vi "GUI_Mlink.vi"() -> ()   [LabVIEW 2020]
uses:
  Shared/GUI_Template/GUI_master/tcp_new_data_event.ctl
  Shared/GUI_Template/GUI_master/tcp new data cluster.ctl
panel:
  in  "Scale":T1(ring)
  in  "trigger::1":enum16{"Internal", "External"}(ring) caption="Trigger"
  in  "stop":bool
  in  "Select device":string(combo)="HPD_EnergyMeter"
  in  "data::1":dbl=25.5 caption="HPD Energy Meter (J)" min=0.0 max=300000000.0 format="%#_6p"
  out "GUIdevice 1":string="HPD_EnergyMeter"
  in  "Clear 2":bool
  out "Ch1":cluster{dbl[], dbl[]}(graph)
  out "Ch1 2":cluster{dbl[], dbl[]}(graph)
  out "tcp data event 2":T2
  out "validdata::1":enum16{"yes", "no"}(ring)
  in  "polarity::1":enum16{"Positive", "Negative"}(ring) caption="Trigger Signal Polarity"
  in  "autorange::1":enum16{"off", "on"}(ring) caption="AutoRange"
  in  "datastream::1":enum16{"off", "on"}(ring)
  in  "insert tag":bool=TRUE
  # "HPD Energy Meter"
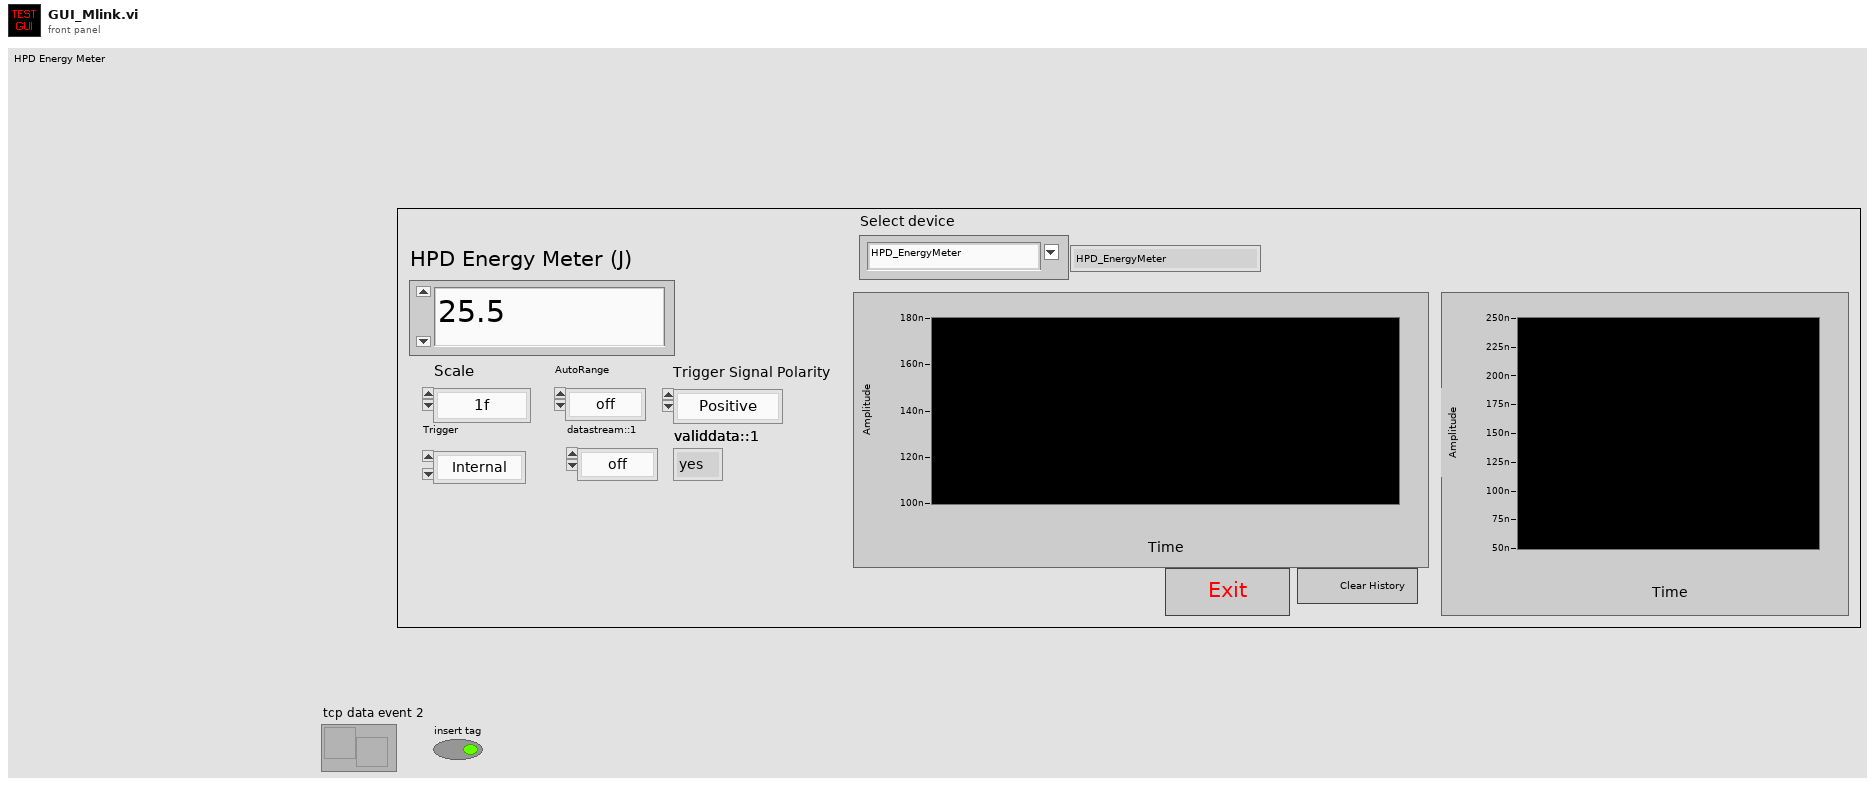
[diagram p1: front panel]
types:
  T1 = enum16{"1f", "3f", "10f", "30f", "100f", "300f", "1p", "3p", "10p", "30p", "100p", "300p", "1n", "3n", "10n", "30n", "100n", "300n", "1u", "3u", "10u", "30u", "100u", "300u", "1m", "3m", "10m", "30m", "100m", "300m", "1", "3", "10", "30", "100", "300", "1K", "3K", "10K", "30K", "100K", "300K", "1M", "3M", "10M", "30M", "100M", "300M"}
  T2 = typedef "tcp_new_data_event.ctl" = refnum<user-event>
  T3 = enum32{"invalid app kind", "Development System", "Run Time System", "Student Edition", "Embedded LabVIEW", "Evaluation", "Custom"}
  T4 = typedef "tcp new data cluster.ctl" = cluster{"EventEnum":enum16{"new data", "connection status update"}, "Device name":string}
  T5 = enum32{"Invalid", "Standard", "Closed", "Hidden", "Minimized", "Maximized"}
  T6 = cluster{"Core":cluster{"Current VI Reference":refnum<vi>, "Close Panel on Exit?":bool}, "Your Boolean data":bool, "Your string data":string, "SuperGUI":cluster{"STOP queue":refnum<queue>, "SuperGUI ref":refnum<vi>, "event reg":refnum<event-registration>}, "Timer":u32}
  T7 = cluster{"STOP queue":refnum<queue>, "SuperGUI ref":refnum<vi>, "event reg":refnum<event-registration>}
  T8 = cluster{"Current VI Reference":refnum<vi>, "Close Panel on Exit?":bool}
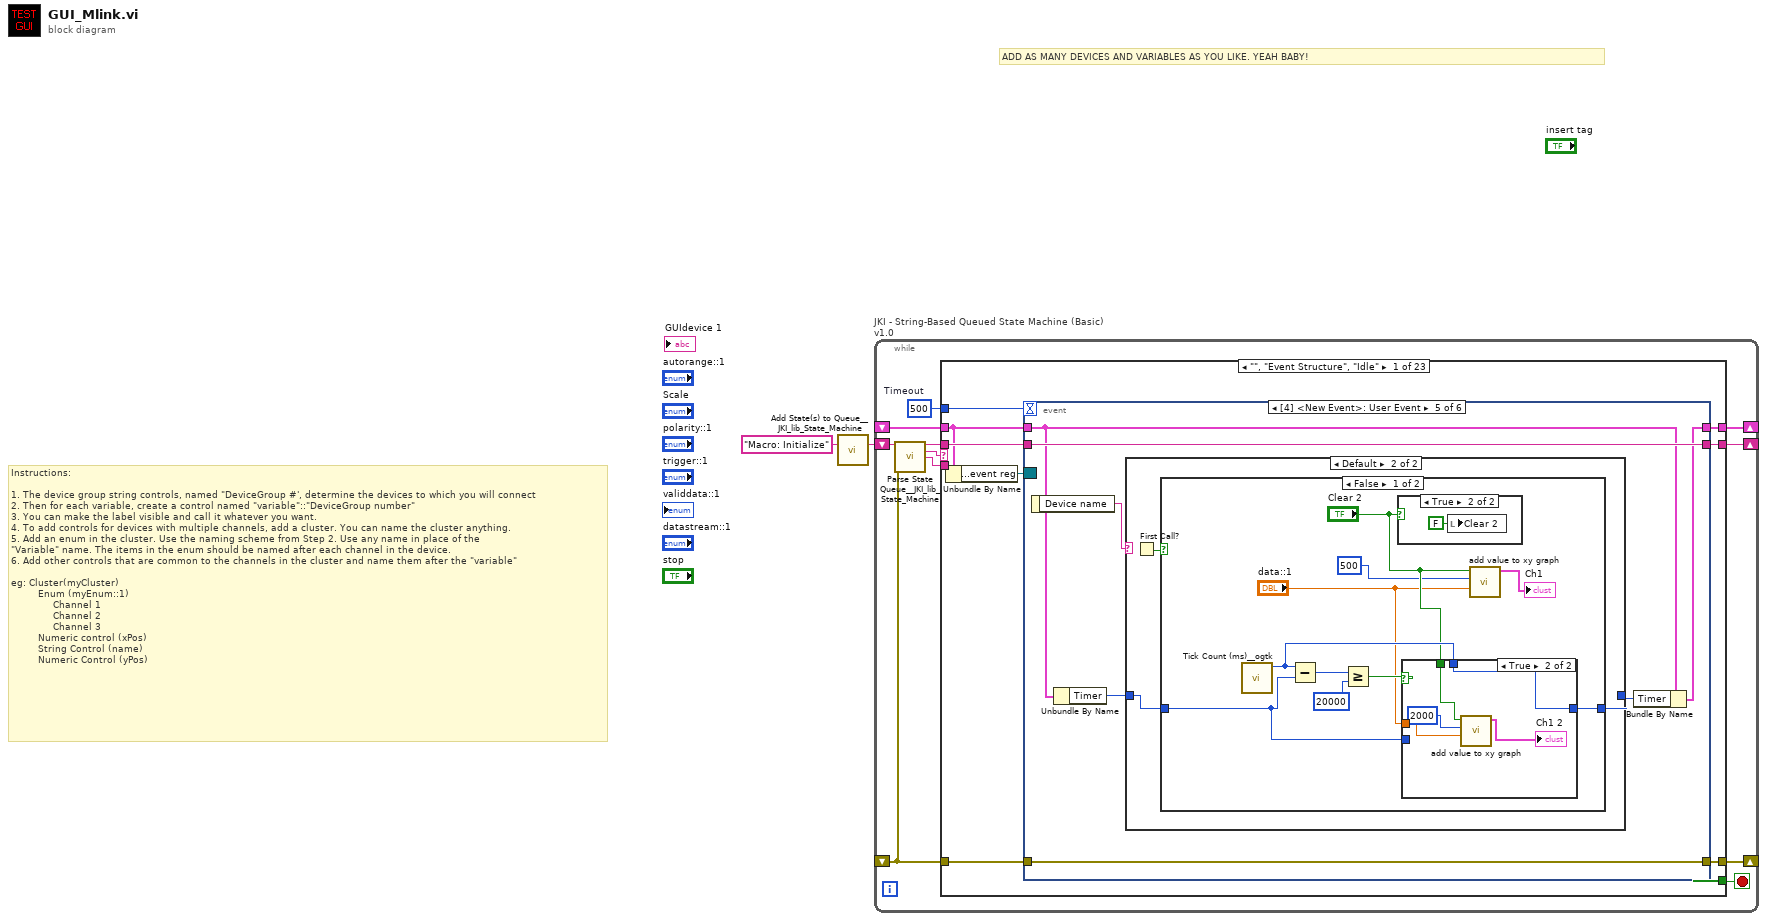
[diagram p0: block diagram]
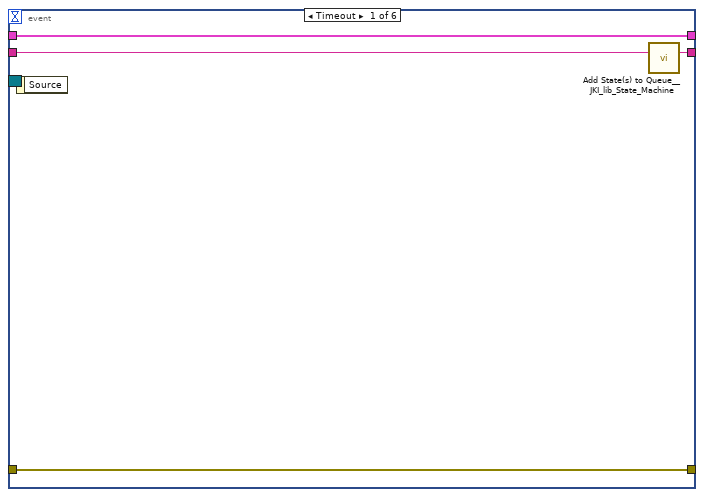
[diagram p2: hidden frame]
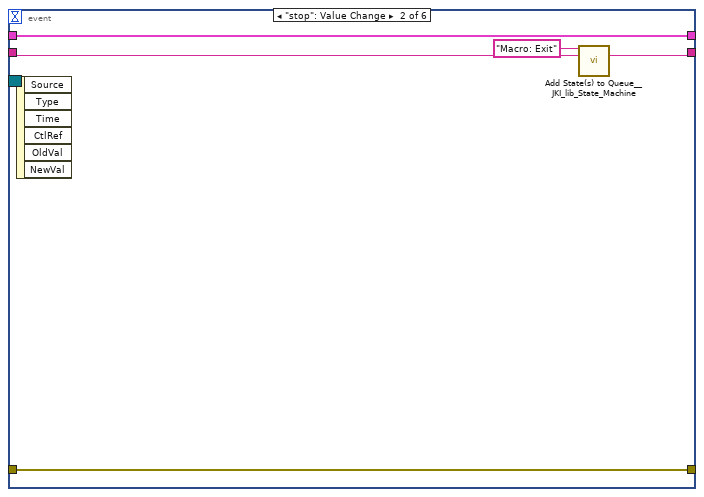
[diagram p3: hidden frame]
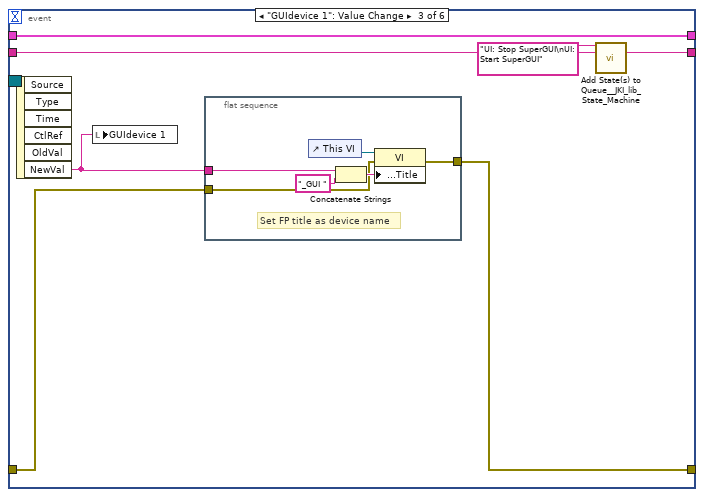
[diagram p4: hidden frame]
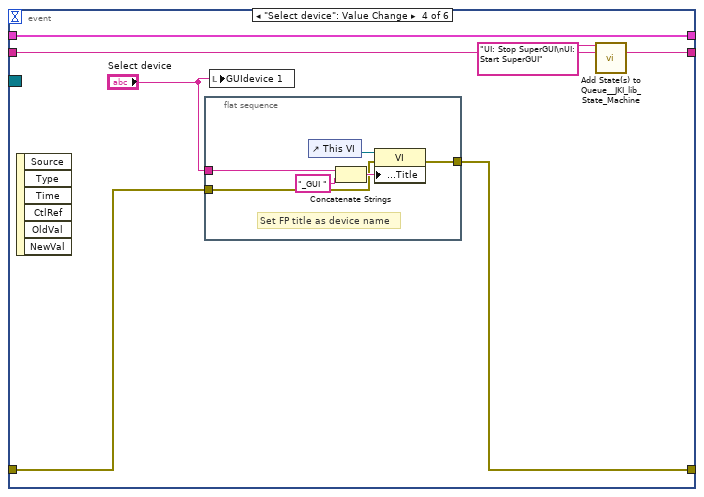
[diagram p5: hidden frame]
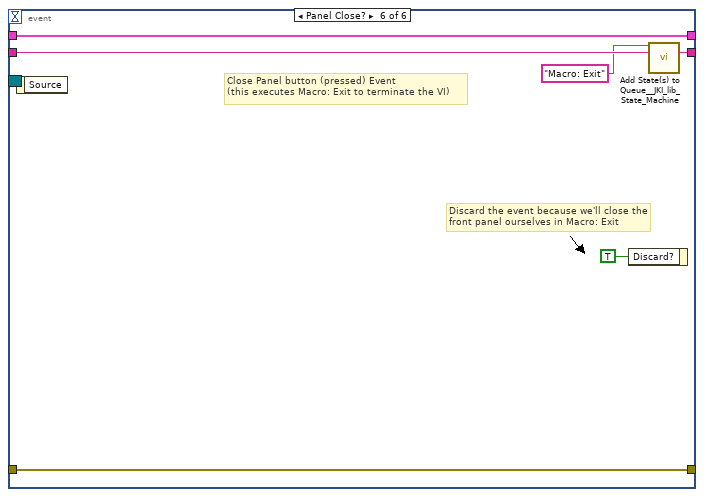
[diagram p10: hidden frame]
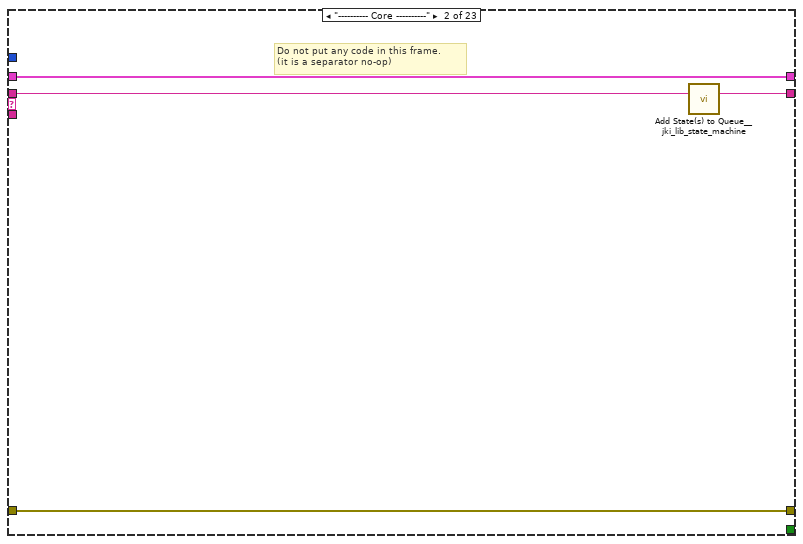
[diagram p11: hidden frame]
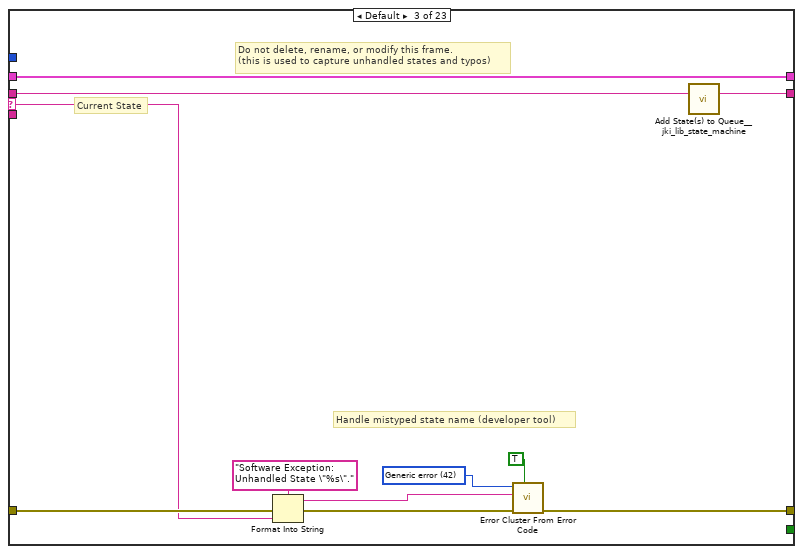
[diagram p12: hidden frame]
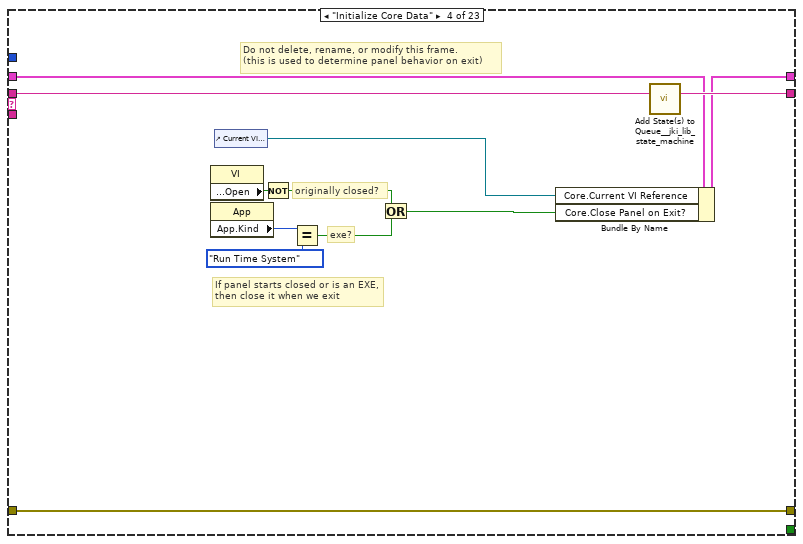
[diagram p13: hidden frame]
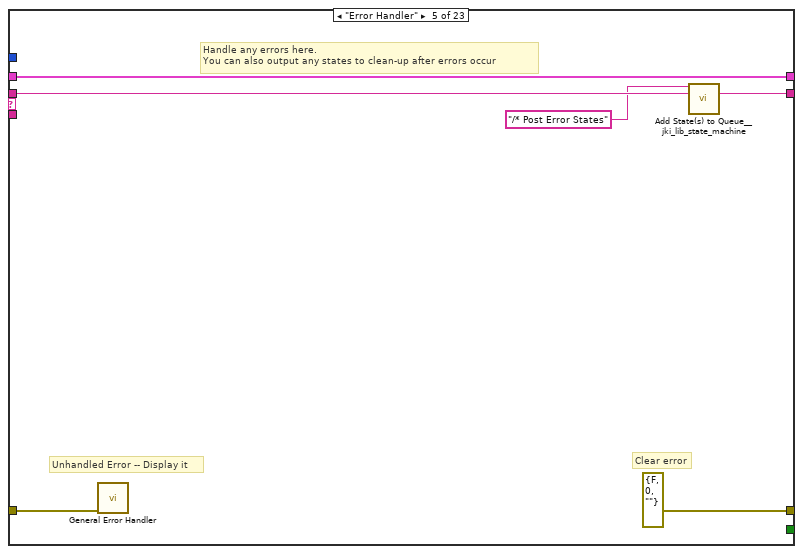
[diagram p14: hidden frame]
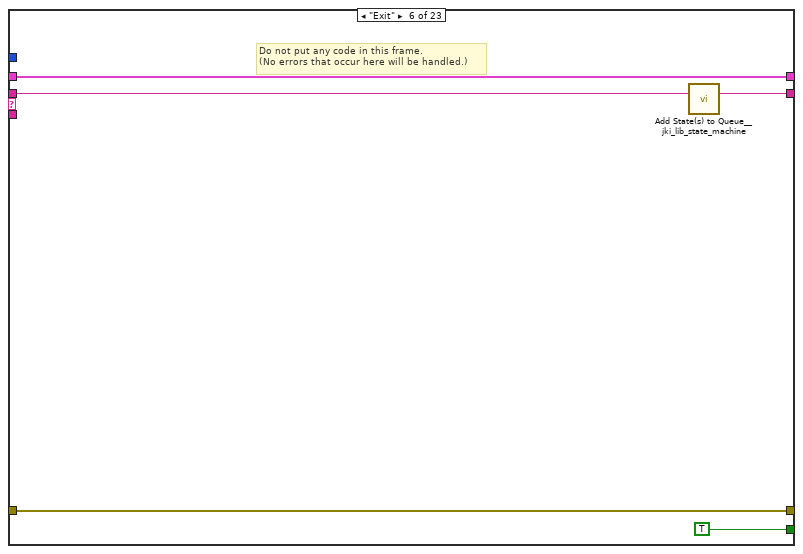
[diagram p15: hidden frame]
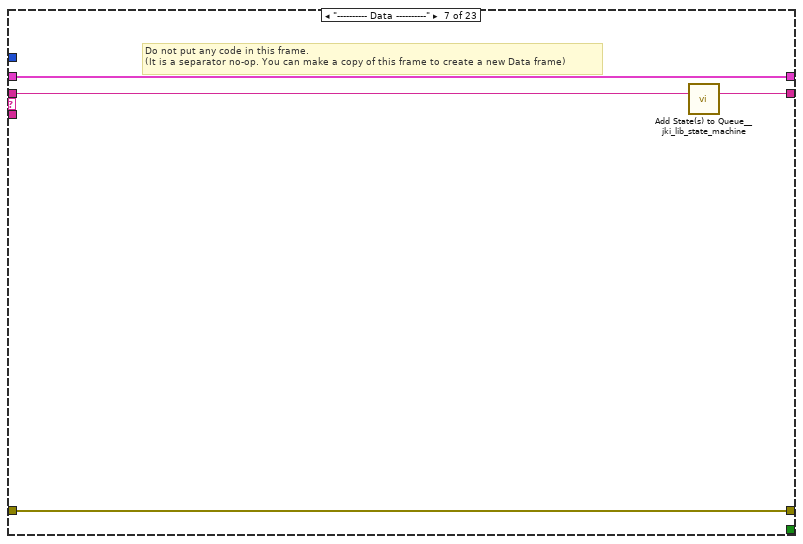
[diagram p16: hidden frame]
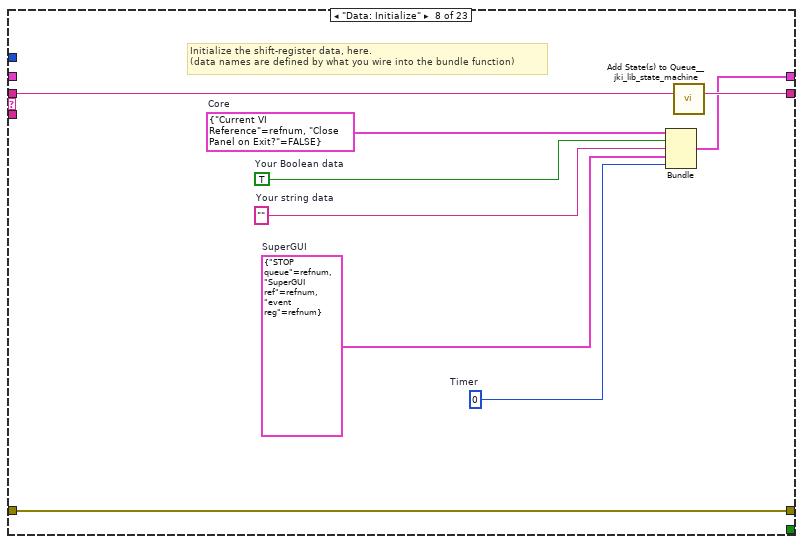
[diagram p17: hidden frame]
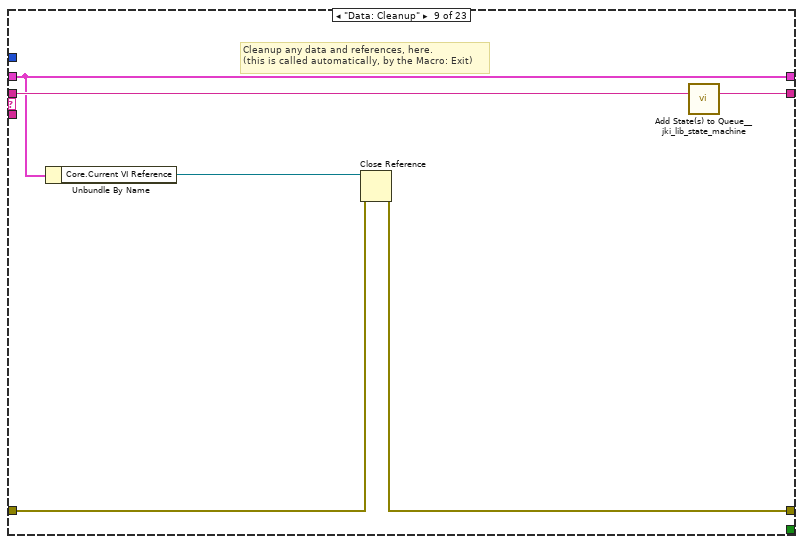
[diagram p18: hidden frame]
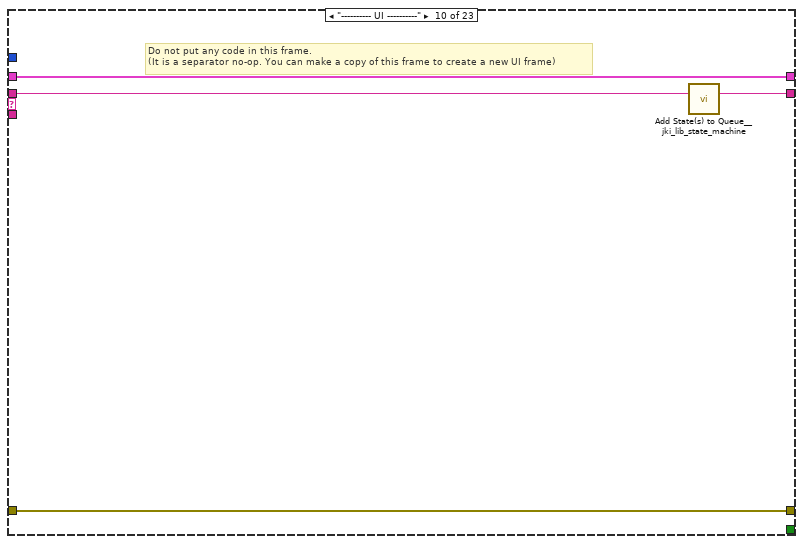
[diagram p19: hidden frame]
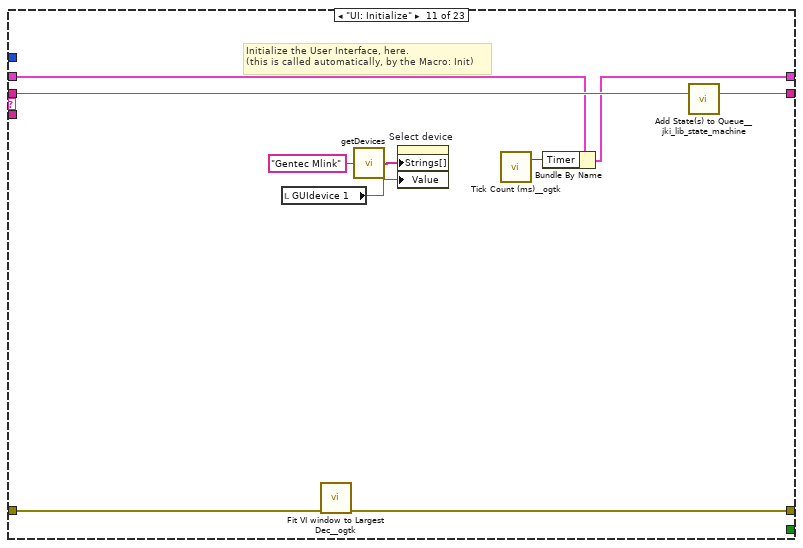
[diagram p20: hidden frame]
diagram:
  # "Instructions:\n\n1. The device group string controls, named \"DeviceGroup #', determine the devices to which you will connect\n2. Then for each variable, create a control named \"variable\"::\"DeviceGroup number\"\n3. You can make the label visible and call it whatever you want.\n4. To add controls for devices with multiple channels, add a cluster. You can name the cluster anything.\n5. Add an enum in the cluster. Use the naming scheme from Step 2. Use any name in place of the \n\"Variable\" name. The items in the enum should be named after each channel in the device. \n6. Add other controls that are common to the channels in the cluster and name them after the \"variable\"\n\neg: Cluster(myCluster)\n         Enum (myEnum::1)\n              Channel 1 \n              Channel 2\n              Channel 3\n         Numeric control (xPos)\n         String Control (name)\n         Numeric Control (yPos)"
  # "ADD AS MANY DEVICES AND VARIABLES AS YOU LIKE. YEAH BABY!"
  n1 = call <vilib>:"Add State(s) to Queue__JKI_lib_State_Machine.vi"("State(s) in (\"\")"="Macro: Initialize") -> ("States Out"=w2:string)  [unwired: 14 in]
  n2 = while "JKI - String-Based Queued State Machine (Basic) v1.0" {
    shift-right: [w6] -> _
    shift-left: _ -> [w5]
    shift-right: [w9] -> _
    shift-left: _ -> [w3]
    shift-right: [w8] -> _
    shift-left: w2 -> [w10]
    stop <- w7 stop-if-true
    w4 = 500  # Timeout
    n3 = call <vilib>:"Parse State Queue__JKI_lib_State_Machine.vi"("State Queue"=w10, "Error In (no error)"=w3) -> ("Remaining States"=w12:string, "Current State"=w13:string, "Arguments"=w11:string)  [unwired: 11 in]
    n4 = case shown="\"\", \"Event Structure\", \"Idle\"" w13 {
      selector: w13 -> [_ _ w96 _ _ _ _ _ _ _ _ _ _ _ _ _ _ _ _ _ _ _ _]
      tunnel: w12 -> [w21 w95 w100 w118 w124 w129 w133 w142 w148 w152 w162 w166 w172 w207 w215 w221 w232 w258 w263 w273 w277 w281 w285]
      tunnel: w11 -> [_ _ _ _ _ _ _ _ _ _ _ _ _ _ _ w216 w226 _ _ _ _ _ _]
      tunnel: w5 -> [w15 w92 w98 w109 w121 w127 w130 _ w143 w149 w155 w164 w170 w198 w210 w219 w228 w255 w260 w270 w274 w278 w282]
      tunnel: [w19 w93 w102 w115 errorcluster {"status"=FALSE, "code"=0, "source"=""} ("error out") w126 w131 w139 w144 w150 w159 w163 w167 w191 w208 w217 w229 w256 w261 w271 w275 w279 w283] -> w9
      tunnel: w3 -> [w18 w93 w101 w115 w120 w126 w131 w139 w145 w150 w160 w163 w168 w192 w209 w218 w230 w256 w261 w271 w275 w279 w283]
      tunnel: [w20 w94 w99 w117 w123 w128 w132 w141 w147 w151 w161 w165 w171 w206 w214 w220 w231 w257 w262 w272 w276 w280 w284] -> w8
      tunnel: [_ _ _ _ _ TRUE _ _ _ _ _ _ _ _ _ _ _ _ _ _ _ _ _] -> w7
      tunnel: [w17 w92 w98 w116 w121 w127 w130 w140 w143 w149 w154 w164 w170 w197 w210 w219 w228 w255 w260 w270 w274 w278 w282] -> w6
      tunnel: w4 -> [w16 _ _ _ _ _ _ _ _ _ _ _ _ _ _ _ _ _ _ _ _ _ _]
      frame "", "Event Structure", "Idle" {
        n5 = Unbundle By Name(w15) -> ("SuperGUI.event reg"=w14:refnum<event-registration>)
        n6 = event shown="[4] <New Event>: User Event" {
          selector: w14 -> [_ _ _ _ _ _]
          dyn-events: _ -> [_ _ _ _ _ _]
          timeout: w16 -> [_ _ _ _ _ _]
          tunnel: w21 -> [w25 w28 w34 w47 w63 w91]
          tunnel: [w24 w27 w33 w46 w63 w90] -> w20
          tunnel: w15 -> [w22 w30 w37 w50 w59 w88]
          tunnel: [w23 w29 w35 w48 w62 w89] -> w19
          tunnel: w18 -> [w23 w29 w36 w49 w62 w89]
          tunnel: [w22 w30 w37 w50 w58 w88] -> w17
          event Timeout {
            n7 = event-data() -> ()  [unwired: 1 in, 1 out]
            n8 = call <vilib>:"Add State(s) to Queue__JKI_lib_State_Machine.vi"("State(s) in (\"\")"=w25) -> ("States Out"=w24:string)  [unwired: 14 in]
          }
          event "stop": Value Change {
            n9 = event-data() -> ()  [unwired: 1 in, 6 out]
            n10 = call <vilib>:"Add State(s) to Queue__JKI_lib_State_Machine.vi"("State(s) in Front (\"\")"="Macro: Exit", "State(s) in (\"\")"=w28) -> ("States Out"=w27:string)  [unwired: 13 in]
          }
          event "GUIdevice 1": Value Change {
            n11 = event-data() -> ("NewVal"=w31:string)  [unwired: 1 in, 5 out]
            n12 = local write "GUIdevice 1"(w31) -> ()
            n13 = flat-sequence {
              tunnel: [w40] -> w35
              tunnel: w36 -> [w39]
              tunnel: w31 -> [w38]
              frame #0 {
                # "Set FP title as device name"
                n14 = control-ref of="This VI"() -> (w43:refnum<vi>)
                n15 = Concatenate Strings(w38, "_GUI ") -> (w42:string)
                n16 = property class="VI"(reference=w43, error in=w39, "Front Panel.Title"=w42) -> (error out=w40:errorcluster)  [unwired: 1 out]
              }
            }
            n17 = call <vilib>:"Add State(s) to Queue__JKI_lib_State_Machine.vi"("State(s) in Front (\"\")"="UI: Stop SuperGUI\nUI: Start SuperGUI", "State(s) in (\"\")"=w34) -> ("States Out"=w33:string)  [unwired: 13 in]
          }
          event "Select device": Value Change {
            n18 = event-data() -> ()  [unwired: 1 in, 6 out]
            n19 = flat-sequence {
              tunnel: [w53] -> w48
              tunnel: w49 -> [w52]
              tunnel: "Select device" -> [w51]
              frame #0 {
                # "Set FP title as device name"
                n20 = control-ref of="This VI"() -> (w56:refnum<vi>)
                n21 = Concatenate Strings(w51, "_GUI ") -> (w55:string)
                n22 = property class="VI"(reference=w56, error in=w52, "Front Panel.Title"=w55) -> (error out=w53:errorcluster)  [unwired: 1 out]
              }
            }
            n23 = local write "GUIdevice 1"("Select device") -> ()
            n24 = call <vilib>:"Add State(s) to Queue__JKI_lib_State_Machine.vi"("State(s) in Front (\"\")"="UI: Stop SuperGUI\nUI: Start SuperGUI", "State(s) in (\"\")"=w47) -> ("States Out"=w46:string)  [unwired: 13 in]
          }
          event User Event {
            n25 = event-data() -> ("Device name"=w60:string)  [unwired: 1 in]
            n26 = Unbundle By Name(w59) -> ("Timer"=w61:u32)
            n27 = case shown="Default" w60 {
              tunnel: w61 -> [w64 w65]
              tunnel: [w64 w66] -> w57
              frame "" {
              }
              frame Default {
                n28 = First Call?() -> (First Call?: T/F=w67:bool)
                n29 = case shown="False" w67 {
                  tunnel: w65 -> [w72 w85]
                  tunnel: [w74 w85] -> w66
                  frame False {
                    n30 = call <userlib>:"Tick Count (ms)__ogtk.vi"() -> ("millisecond timer value"=w73:u32)  [unwired: 10 in, 1 out]
                    n31 = Subtract(x=w73, y=w72) -> (x-y=w76:u32)
                    n32 = Greater Or Equal?(x=w76, y=u32 20000 ("min time between updates")) -> (x >= y?=w75:bool)
                    n33 = case shown="True" "Clear 2" {
                      frame False {
                      }
                      frame True {
                        n34 = local write "Clear 2"(FALSE ("Clear")) -> ()
                      }
                    }
                    n35 = case shown="True" w75 {
                      tunnel: "data::1" -> [_ w81]
                      tunnel: [w78 w83] -> w74
                      tunnel: w73 -> [_ w83]
                      tunnel: w72 -> [w78 _]
                      tunnel: "Clear 2" -> [_ w79]
                      frame False {
                      }
                      frame True {
                        n36 = call "add value to xy graph.vi"("new value"=w81, "max points"=2000, "Wire in Stop To Clear Graph on Each Run"=w79) -> ("XY Graph"=→"Ch1 2":cluster{dbl[], dbl[]})  [unwired: 8 in]
                      }
                    }
                    n37 = call "add value to xy graph.vi"("new value"="data::1", "max points"=500, "Wire in Stop To Clear Graph on Each Run"="Clear 2") -> ("XY Graph"=→"Ch1":cluster{dbl[], dbl[]})  [unwired: 8 in]
                  }
                  frame True {
                  }
                }
              }
            }
            n38 = Bundle By Name(cluster=w59, "Timer"=w57) -> (w58:T6)
          }
          event Panel Close? {
            # "Discard the event because we'll close the front panel ourselves in Macro: Exit"
            # "Close Panel button (pressed) Event\n(this executes Macro: Exit to terminate the VI)"
            n39 = event-data() -> ()  [unwired: 1 in, 1 out]
            n40 = event-data("Discard?"=TRUE) -> ()  [unwired: 1 in, 1 out]
            n41 = call <vilib>:"Add State(s) to Queue__JKI_lib_State_Machine.vi"("State(s) in Front (\"\")"="Macro: Exit", "State(s) in (\"\")"=w91) -> ("States Out"=w90:string)  [unwired: 13 in]
          }
        }
      }
      frame "---------- Core ----------" {
        # "Do not put any code in this frame.\n(it is a separator no-op)"
        n42 = call <vilib>:"Add State(s) to Queue__jki_lib_state_machine.vi"("State(s) in (\"\")"=w95) -> ("States Out"=w94:string)  [unwired: 14 in]
      }
      frame Default {
        w105 = 42 items=["No error", "Argument error", "Memory is full", "Out of zone", "End of file", "File already open", "Generic file I/O error", "File not found", "File permission error", "Disk is full", "Duplicate path", "Too many files open", "System feature not enabled", "Resource file not found", "Cannot add resource", "Resource not found", "Image not found", "Image memory error", "Pen does not exist", "Config type invalid", "Config token not found", "Config parse error", "Config memory error", "Bad external code format", "Bad external code offset", "External code not present", "Null window", "Destroy window error", "Null menu", "Print aborted", "Bad print record", "Print driver error", "Windows error during printing", "Memory error during printing", "Print dialog error", "Generic print error", "Invalid device refnum", "Device not found", "Device parameter error", "Device unit error", "Cannot open device", "Device call aborted", "Generic error", "Cancelled by user", "Object ID too low", "Object ID too high", "Object not in heap", "Unknown heap", "Unknown object (invalid DefProc)", "Unknown object (DefProc not in table)", "Message out of range", "Invalid (null) method", "Unknown message", "Manager call not supported", "Bad address", "Network operation in progress", "Network operation timed out", "Connection is busy", "Network attribute not supported", "Network error", "Address in use", "System out of memory", "Connection aborted", "Connection refused", "Not connected", "Already connected", "Connection closed", "Initialization error (interapplication manager)", "Bad occurrence", "Wait on unbound occurrence handler", "Occurrence queue overflow", "Datalog type conflict", "Unused", "Unrecognized type (interapplication manager)", "Memory corrupt", "Failed to make temporary DLL", "Old CIN version", "Drag socket not found", "Failed to load drop-object", "Failed to register OLE object", "Failed to release OLE object", "Format specifier type mismatch", "Unknown format specifier", "Too few format specifiers", "Too many format specifiers", "Scan failed", "Newer CIN version", "Error converting to variant", "Runtime menu error", "Password tampered", "Variant attribute not found", "Incompatible variant data type", "Event data is not available", "Event Store is not present", "Occurrence is not found", "Event Queue is not created", "Event info is not available", "Refnum passed is NULL", "Error retrieving Class GUID", "Error retrieving CoClass GUID", "Error retrieving TypeLib GUID.", "Bad built application magic bytes.", "Specific driver is different from the specific driver associated with the Logical Name.", "There is no session opened to the class driver.", "Max Error", "MAX - Error with config objects", "MAX - Error loading configuration", "MAX - Group not supported"]
        # "Current State"
        # "Do not delete, rename, or modify this frame.\n(this is used to capture unhandled states and typos)"
        # "Handle mistyped state name (developer tool)"
        n43 = Format Into String(format string="Software Exception: Unhandled State \"%s\"." ("message"), error in=w101, w96) -> (resulting string=w104:string, error out=w103:errorcluster)  [unwired: 1 in]
        n44 = call <vilib>:"Error Cluster From Error Code.vi"("show call chain? (False)"=TRUE, "error in (no error)"=w103, "error message (\"\")"=w104, "error code (0)"=w105) -> ("error out"=w102:errorcluster)  [unwired: 5 in]
        n45 = call <vilib>:"Add State(s) to Queue__jki_lib_state_machine.vi"("State(s) in (\"\")"=w100) -> ("States Out"=w99:string)  [unwired: 14 in]
      }
      frame "Initialize Core Data" {
        # "Do not delete, rename, or modify this frame.\n(this is used to determine panel behavior on exit)"
        # "originally closed?"
        # "exe?"
        # "If panel starts closed or is an EXE, then close it when we exit"
        n46 = property class="VI"() -> ("Front Panel.Open"=w114:bool)  [unwired: 2 in, 2 out]
        n47 = property class="App"() -> ("App.Kind"=w113:T3)  [unwired: 2 in, 2 out]
        n48 = control-ref of="Current VI Reference"() -> (w107:refnum<vi>)
        n49 = Not(x=w114) -> (.not. x?=w111:bool)
        n50 = Equal?(x=w113, y=T3."Run Time System" ("Application:Kind")) -> (x = y?=w110:bool)
        n51 = Or(x=w111, y=w110) -> (x .or. y?=w108:bool)
        n52 = Bundle By Name(cluster=w109, "Core.Current VI Reference"=w107, "Core.Close Panel on Exit?"=w108) -> (w116:T6)
        n53 = call <vilib>:"Add State(s) to Queue__jki_lib_state_machine.vi"("State(s) in (\"\")"=w118) -> ("States Out"=w117:string)  [unwired: 14 in]
      }
      frame "Error Handler" {
        # "Unhandled Error -- Display it"
        # "Handle any errors here.\nYou can also output any states to clean-up after errors occur"
        # "Clear error"
        n54 = call <vilib>:"General Error Handler.vi"("error in (no error)"=w120) -> ()  [unwired: 10 in, 5 out]
        n55 = call <vilib>:"Add State(s) to Queue__jki_lib_state_machine.vi"("State(s) in Front (\"\")"="/* Post Error States", "State(s) in (\"\")"=w124) -> ("States Out"=w123:string)  [unwired: 13 in]
      }
      frame "Exit" {
        # "Do not put any code in this frame.\n(No errors that occur here will be handled.)"
        n56 = call <vilib>:"Add State(s) to Queue__jki_lib_state_machine.vi"("State(s) in (\"\")"=w129) -> ("States Out"=w128:string)  [unwired: 14 in]
      }
      frame "---------- Data ----------" {
        # "Do not put any code in this frame.\n(It is a separator no-op. You can make a copy of this frame to create a new Data frame)"
        n57 = call <vilib>:"Add State(s) to Queue__jki_lib_state_machine.vi"("State(s) in (\"\")"=w133) -> ("States Out"=w132:string)  [unwired: 14 in]
      }
      frame "Data: Initialize" {
        w134 = u32 0  # Timer
        w135 = T7 {"STOP queue"=refnum, "SuperGUI ref"=refnum, "event reg"=refnum}  # SuperGUI
        w136 = T8 {"Current VI Reference"=refnum, "Close Panel on Exit?"=FALSE}  # Core
        w138 = TRUE  # Your Boolean data
        w137 = ""  # Your string data
        # "Initialize the shift-register data, here.\n(data names are defined by what you wire into the bundle function)"
        n58 = Bundle("Core"=w136, "Your Boolean data"=w138, "Your string data"=w137, "SuperGUI"=w135, "Timer"=w134) -> (w140:T6)  [unwired: 1 in]
        n59 = call <vilib>:"Add State(s) to Queue__jki_lib_state_machine.vi"("State(s) in (\"\")"=w142) -> ("States Out"=w141:string)  [unwired: 14 in]
      }
      frame "Data: Cleanup" {
        # "Cleanup any data and references, here.\n(this is called automatically, by the Macro: Exit)"
        n60 = Unbundle By Name(w143) -> ("Core.Current VI Reference"=w146:refnum<vi>)
        n61 = Close Reference(reference=w146, error in (no error)=w145) -> (error out=w144:errorcluster)
        n62 = call <vilib>:"Add State(s) to Queue__jki_lib_state_machine.vi"("State(s) in (\"\")"=w148) -> ("States Out"=w147:string)  [unwired: 14 in]
      }
      frame "---------- UI ----------" {
        # "Do not put any code in this frame.\n(It is a separator no-op. You can make a copy of this frame to create a new UI frame)"
        n63 = call <vilib>:"Add State(s) to Queue__jki_lib_state_machine.vi"("State(s) in (\"\")"=w152) -> ("States Out"=w151:string)  [unwired: 14 in]
      }
      frame "UI: Initialize" {
        # "Initialize the User Interface, here.\n(this is called automatically, by the Macro: Init)"
        n64 = local read "GUIdevice 1"() -> (w156:string)
        n65 = call <userlib>:"Fit VI window to Largest Dec__ogtk.vi"("error in (no error)"=w160) -> ("error out"=w159:errorcluster)  [unwired: 5 in, 1 out]
        n66 = call "getDevices.vi"("Device Class"="Gentec Mlink") -> ("All Devices"=w158:string[])
        n67 = property on="Select device" class="CmbBox"("Strings[]"=w158, "Value"=w156) -> ()  [unwired: 2 in, 2 out]
        n68 = call <userlib>:"Tick Count (ms)__ogtk.vi"() -> ("millisecond timer value"=w153:u32)  [unwired: 10 in, 1 out]
        n69 = Bundle By Name(cluster=w155, "Timer"=w153) -> (w154:T6)
        n70 = call <vilib>:"Add State(s) to Queue__jki_lib_state_machine.vi"("State(s) in (\"\")"=w162) -> ("States Out"=w161:string)  [unwired: 14 in]
      }
      frame "UI: Update Device List" {
        n71 = call <vilib>:"Add State(s) to Queue__jki_lib_state_machine.vi"("State(s) in (\"\")"=w166) -> ("States Out"=w165:string)  [unwired: 14 in]
      }
      frame "UI: Get Device Name" {
        n72 = First Call?() -> (First Call?: T/F=w169:bool)
        n73 = case shown="True" w169 {
          tunnel: w168 -> [w173 w175]
          tunnel: [w173 w174] -> w167
          frame False {
          }
          frame True {
            n74 = disable-structure "Get Device name from control for vi mode\nand command line arg for exe" shown="RUN_TIME_ENGINE==True" {
              disable-tunnel: w175 -> [_ w177]
              disable-tunnel: [_ w176] -> w174
              frame condition #0 (active) {
              }
              frame condition #1 {
                n75 = control-ref of="This Application"() -> (w185:refnum<vi>)
                n76 = property class="App"(reference=w185) -> ("App.Args"=w184:string[])  [unwired: 1 in, 2 out]
                n77 = Index Array(array=w184, index #1=1 ("index")) -> (element #1=w178:string)  [unwired: 2 in, 2 out]
                n78 = Empty String/Path?(string/path=w178) -> (empty?=w182:bool)
                n79 = control-ref of="This VI"() -> (w181:refnum<vi>)
                n80 = case shown="False" w182 {
                  tunnel: w178 -> [w186 _]
                  frame False {
                    n81 = local write "GUIdevice 1"(w186) -> ()
                  }
                  frame True {
                  }
                }
                n82 = Concatenate Strings(w178, "_GUI ") -> (w180:string)
                n83 = property class="VI"(reference=w181, error in=w177, "Front Panel.Title"=w180) -> (error out=w176:errorcluster)  [unwired: 1 out]
              }
            }
          }
        }
        n84 = call <vilib>:"Add State(s) to Queue__jki_lib_state_machine.vi"("State(s) in (\"\")"=w172) -> ("States Out"=w171:string)  [unwired: 14 in]
      }
      frame "UI: Start SuperGUI" {
        # "create stop queue for supergui and its clones"
        # "x100 abort will be dependent on caller VI\nx80 abort will be independent of caller vi, this will abort vi when labview is closed."
        # "Start SuperGUI asynchronous way"
        n85 = vi-ref "GUI_Master_subvi_reentrant_queues.vi"() -> (w190:refnum<vi>)
        n86 = property class="VI"(reference=w190) -> ("Path"=w189:path)  [unwired: 1 in, 2 out]
        n87 = Create User Event(user event datatype=T4 {"EventEnum"=enum."new data", "Device name"="Device name"} ("New Event"), error in=w192) -> (user event=w193:refnum<user-event>, error out=w199:errorcluster)
        "tcp data event 2" <- w193
        n88 = control-ref of="This Application"() -> (w196:refnum<vi>)
        n89 = control-ref of="This VI"() -> (w195:refnum<vi>)
        n90 = Open VI Reference(type specifier VI Refnum (for type only)=refnum<vi> refnum, vi path=w189, options=256) -> (vi reference=w205:refnum<vi>, error out=w204:errorcluster)  [unwired: 3 in]
        n91 = register-events(w193) -> (reference out=w187:refnum<event-registration>)  [unwired: 2 in, 1 out]
        n92 = call "supergui create stop queue.vi"() -> ("STOP Queue out"=w201:refnum<queue>)  [unwired: 11 in]
        n93 = Current VI's Menubar() -> (w194:refnum<k9>)
        n94 = call-by-ref "Start Asynchronous Call"(reference=w205, error in=w204, "STOP Queue in"=w201, "This Application"=w196, 8:"error in (no error)"=w199, "tcp data event"=w193, "Caller menu reference"=w194, "Caller VI ref"=w195) -> (reference out=w188:refnum<vi>, error out=w191:errorcluster)  [unwired: 5 in, 1 out]
        n95 = Bundle By Name(cluster=w198, "SuperGUI.event reg"=w187, "SuperGUI.SuperGUI ref"=w188, "SuperGUI.STOP queue"=w201) -> (w197:T6)
        n96 = call <vilib>:"Add State(s) to Queue__jki_lib_state_machine.vi"("State(s) in (\"\")"=w207) -> ("States Out"=w206:string)  [unwired: 14 in]
      }
      frame "UI: Stop SuperGUI" {
        # "Stop Supergui Clone and wait until it exit properly"
        n97 = Unbundle By Name(w210) -> ("SuperGUI.SuperGUI ref"=w212:refnum<vi>, "SuperGUI.STOP queue"=w211:refnum<queue>)
        n98 = Release Queue(queue=w211, error in (no error)=w209) -> (error out=w213:errorcluster)  [unwired: 1 in, 2 out]
        n99 = call-by-ref "Wait On Asynchronous Call"(reference=w212, error in=w213) -> ("error out"=w208:errorcluster)  [unwired: 11 in, 2 out]
        n100 = call <vilib>:"Add State(s) to Queue__jki_lib_state_machine.vi"("State(s) in (\"\")"=w215) -> ("States Out"=w214:string)  [unwired: 14 in]
      }
      frame "UI: Cursor Set" {
        # "Argument"
        # "Set and Unset Cursor Busy.\n(Usage: \"UI: Cursor Set >> Busy|Idle\")"
        n101 = case shown="\"Idle\", Default" w216 {
          tunnel: w218 -> [w223 w225]
          tunnel: [w222 w224] -> w217
          frame "Idle", Default {
            n102 = call <vilib>:"Unset Busy.vi"("error in (no error)"=w223) -> ("error out"=w222:errorcluster)  [unwired: 10 in]
          }
          frame "Busy" {
            n103 = call <vilib>:"Set Busy.vi"("error in (no error)"=w225) -> ("error out"=w224:errorcluster)  [unwired: 9 in, 1 out]
          }
        }
        n104 = call <vilib>:"Add State(s) to Queue__jki_lib_state_machine.vi"("State(s) in (\"\")"=w221) -> ("States Out"=w220:string)  [unwired: 14 in]
      }
      frame "UI: Front Panel State" {
        # "Argument"
        # "Set Front Panel Open or Closed\n(Usage: \"UI: Front Panel State >> Open|Close\")"
        n105 = Unbundle By Name(w228) -> ("Core.Current VI Reference"=w227:refnum<vi>)
        n106 = case shown="\"Open\", Default" w226 {
          tunnel: w230 -> [w236 w249]
          tunnel: [w238 w250] -> w229
          tunnel: w227 -> [w237 w247]
          frame "Open", Default {
            n107 = property class="VI"(reference=w237, error in=w236) -> (reference out=w234:refnum<vi>, error out=w235:errorcluster, "Front Panel.Open"=w233:bool)
            n108 = case shown="False" w233 {
              tunnel: [w241 w244] -> w238
              tunnel: w235 -> [w240 w244]
              tunnel: w234 -> [w239 _]
              frame False {
                n109 = invoke class="VI" method="FP.Open"(reference=w239, error in=w240, "Activate"=TRUE, "State"=T5."Standard") -> (error out=w241:errorcluster)  [unwired: 1 in, 4 out]
              }
              frame True {
              }
            }
          }
          frame "Close" {
            n110 = property class="VI"(reference=w247, error in=w249) -> (reference out=w246:refnum<vi>, error out=w248:errorcluster, "Front Panel.Open"=w245:bool)
            n111 = case shown="True" w245 {
              tunnel: [w251 w254] -> w250
              tunnel: w248 -> [w251 w253]
              tunnel: w246 -> [_ w252]
              frame False {
              }
              frame True {
                n112 = invoke class="VI" method="FP.Close"(reference=w252, error in=w253) -> (error out=w254:errorcluster)  [unwired: 1 in, 2 out]
              }
            }
          }
        }
        n113 = call <vilib>:"Add State(s) to Queue__jki_lib_state_machine.vi"("State(s) in (\"\")"=w232) -> ("States Out"=w231:string)  [unwired: 14 in]
      }
      frame "---------- Macro ----------" {
        # "Do not put any code in this frame.\n(It is a separator no-op. You can make a copy of this frame to create a new Macro frame)"
        n114 = call <vilib>:"Add State(s) to Queue__jki_lib_state_machine.vi"("State(s) in (\"\")"=w258) -> ("States Out"=w257:string)  [unwired: 14 in]
      }
      frame "Macro: Initialize" {
        # "Initialization Macro\n(This is called once, when the VI starts)"
        n115 = call <vilib>:"Add State(s) to Queue__jki_lib_state_machine.vi"("State(s) in Front (\"\")"="Data: Initialize\nInitialize Core Data\nUI: Initialize\nUI: Update Device List\nUI: Get Device Name\nUI: Start SuperGUI\nUI: Front Panel State >> Open", "State(s) in (\"\")"=w263) -> ("States Out"=w262:string)  [unwired: 13 in]
      }
      frame "Macro: Exit" {
        # "Exit Macro\n(This is called once, when the VI exits)"
        n116 = Unbundle By Name(w270) -> ("Core.Close Panel on Exit?"=w269:bool)
        n117 = Select(t="UI: Front Panel State >> Close", s=w269, f="") -> (s? t:f=w266:string)
        n118 = call <vilib>:"Add State(s) to Queue__jki_lib_state_machine.vi"("State(s) in (\"\")"=w266, "State(s) at Back (\"\")"="Data: Cleanup\nExit") -> ("States Out"=w264:string)  [unwired: 13 in]
        n119 = call <vilib>:"Add State(s) to Queue__jki_lib_state_machine.vi"("State(s) in Front (\"\")"=w264, "State(s) in (\"\")"=w273) -> ("States Out"=w272:string)  [unwired: 13 in]
      }
      frame "---------- New Category ----------" {
        # "Template Separator\n(You can make a copy of, or modify, this frame)"
        n120 = call <vilib>:"Add State(s) to Queue__jki_lib_state_machine.vi"("State(s) in (\"\")"=w277) -> ("States Out"=w276:string)  [unwired: 14 in]
      }
      frame "New Category: 1" {
        # "Your code here.\n(You can make a copy of, or modify, this frame)"
        n121 = call <vilib>:"Add State(s) to Queue__jki_lib_state_machine.vi"("State(s) in (\"\")"=w281) -> ("States Out"=w280:string)  [unwired: 14 in]
      }
      frame "New Category: 2" {
        # "Your code here.\n(You can make a copy of, or modify, this frame)"
        n122 = call <vilib>:"Add State(s) to Queue__jki_lib_state_machine.vi"("State(s) in (\"\")"=w285) -> ("States Out"=w284:string)  [unwired: 14 in]
      }
    }
  }
